vi "get_name_by_CANnodeID.vi"(8 "error in (no error)":errorcluster caption="错误输入（无错误）", 10 "CAN node ID":i32, 11 "MotorSystem 输入":refnum<class "MotorSystem.lvclass">) -> (0 "error out":errorcluster caption="错误输出", 1 "index (0-based)":u32, 2 "name":string, 3 "MotorSystem 输出":refnum<class "MotorSystem.lvclass">)   [LabVIEW 2016, in "MotionControl_UFO_3DOF.lvlib" / "MotorSystem.lvclass"]
uses:
  <userlib>/MotionControl_UFO_3DOF/MotorSystem/MotorSystem.lvclass
  <userlib>/MotionControl_UFO_3DOF/MotorSystem/MotorSystem.lvclass/MotorSystem.ctl
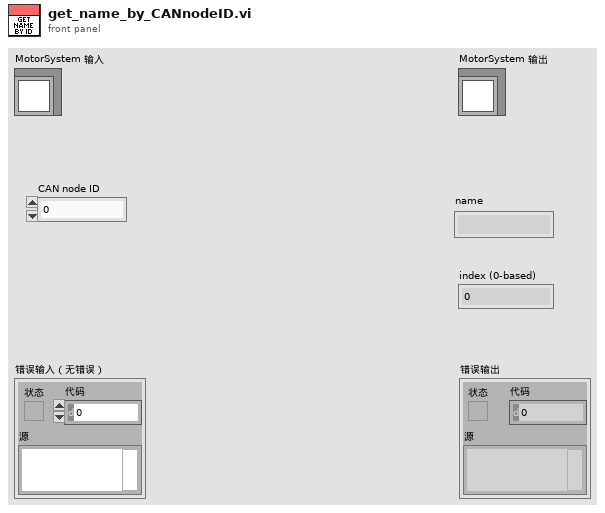
[diagram p1: front panel]
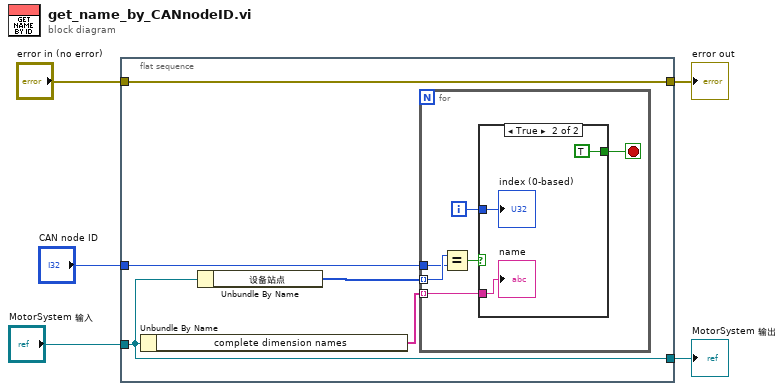
[diagram p0: block diagram]
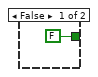
[diagram p2: hidden frame]
diagram:
  n1 = flat-sequence {
    tunnel: "CAN node ID" -> [w9]
    tunnel: "MotorSystem 输入" -> [w7]
    tunnel: [w7] -> w3
    tunnel: "error in (no error)" -> [w6]
    tunnel: [w6] -> w1
    frame #0 {
      n2 = Unbundle By Name(w7) -> ("complete dimension names"=w8:string[])
      n3 = Unbundle By Name(w7) -> ("设备站点"=w10:u32[])
      n4 = for {
        tunnel: w10 -> [w16] mode=indexing
        tunnel: w9 -> [w15]
        tunnel: w8 -> [w13] mode=indexing
        i -> [w11]
        stop <- w12 stop-if-true
        n5 = Equal?(x=w16, y=w15) -> (x = y?=w14:bool)
        n6 = case shown="True" w14 {
          tunnel: w13 -> [_ w20]
          tunnel: [FALSE TRUE] -> w12
          tunnel: w11 -> [_ w18]
          frame False {
          }
          frame True {
            "name" <- w20
            "index (0-based)" <- w18
          }
        }
      }
    }
  }
  "error out" <- w1
  "MotorSystem 输出" <- w3
